vi "_Serial_Mark10-Control (Press Config).vi"(3 "FTS Operation state":T1="Start pressure control", 4 "Press Setting(lb)":dbl=10.0 min=0.0 max=160.0 step=0.01 format="%.2f", 5 "Serial Port":refnum<visa-resource-name>="COM5") -> (0 "Gauge Pressure(lb)":dbl min=0.0 max=160.0 step=0.01 format="%.2f", 1 "Communication is normal":bool=TRUE, 2 "Serial Port out":refnum<visa-resource-name>="COM5")   [LabVIEW 2015]
uses:
  Control-Operation State Mark10.ctl
panel:
  out "Number of fine tuning":u32
  in  "Speed-fine tuning(mm/min)":dbl=1.0
  in  "Speed-Low(mm/min)":dbl=4.0
  in  "Speed-Medium(mm/min)":dbl=60.0
  in  "Speed-High(mm/min)":dbl=250.0
  # "MARK10 Control of Press"
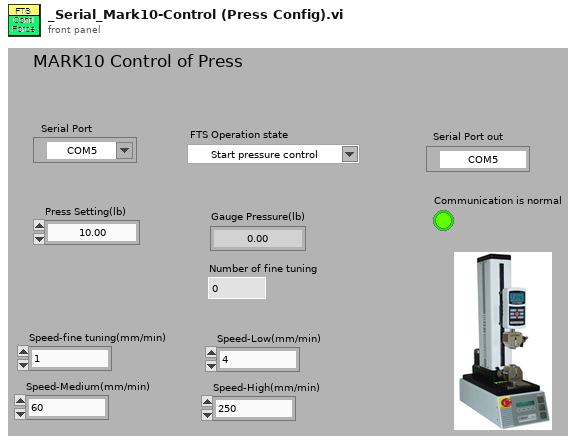
[diagram p1: front panel]
types:
  T1 = typedef "Control-Operation State Mark10.ctl" = string
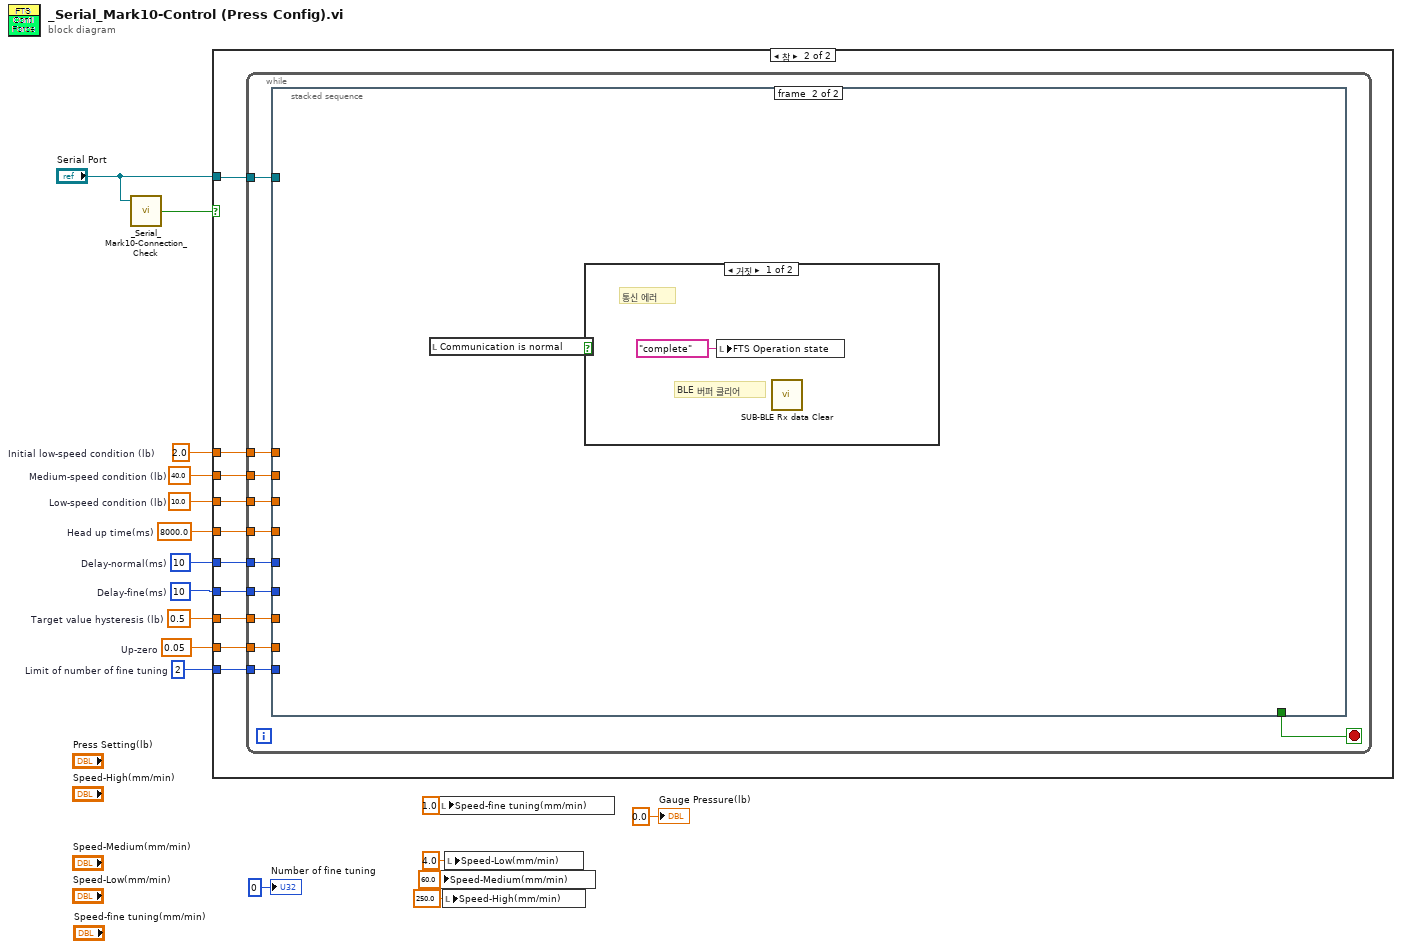
[diagram p0: block diagram]
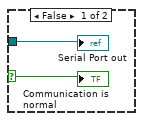
[diagram p2: hidden frame]
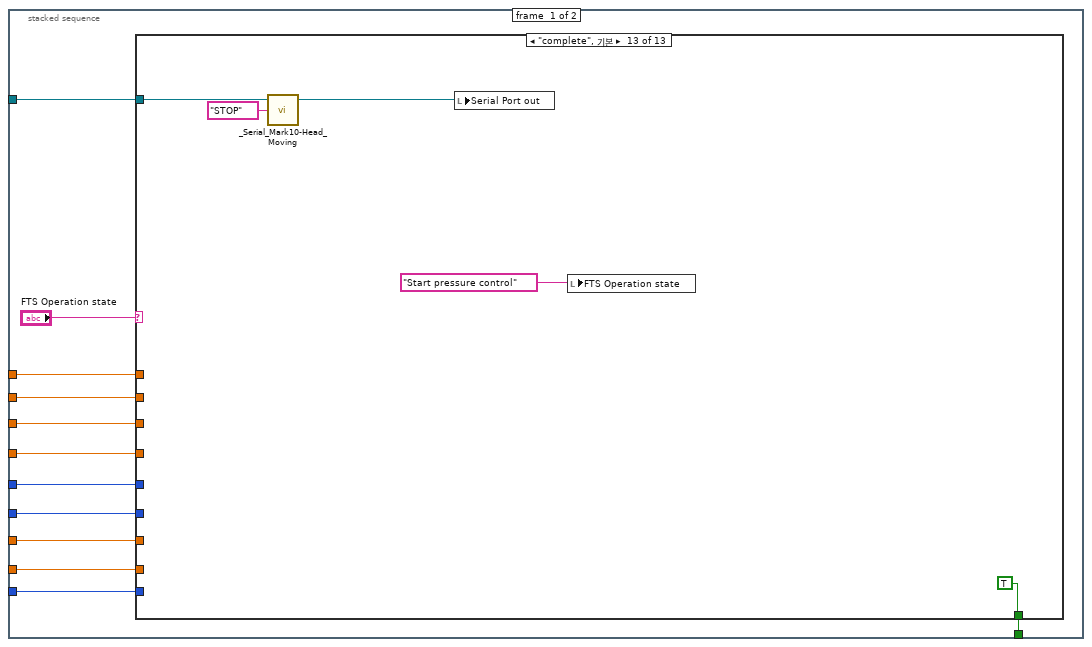
[diagram p3: hidden frame]
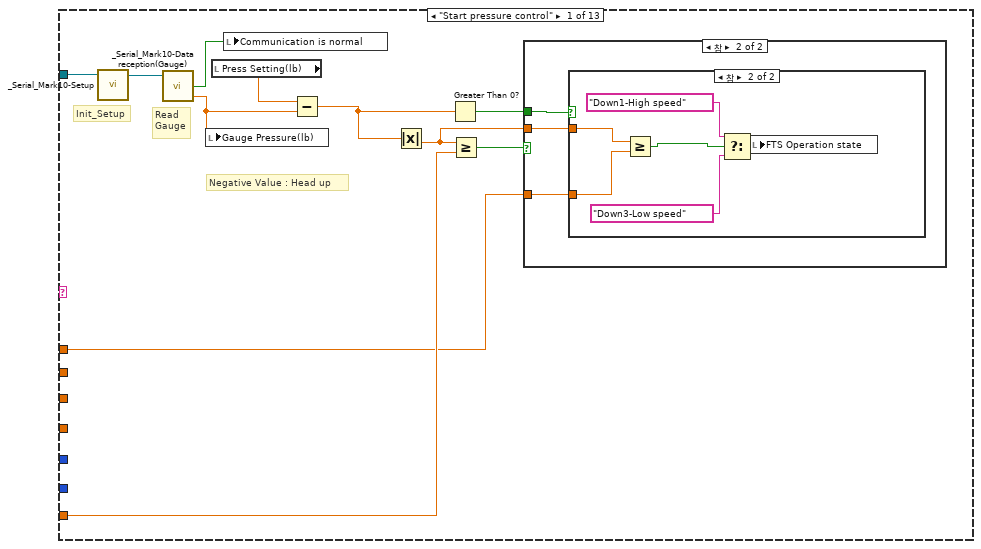
[diagram p4: hidden frame]
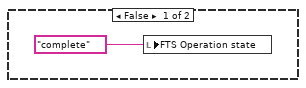
[diagram p5: hidden frame]
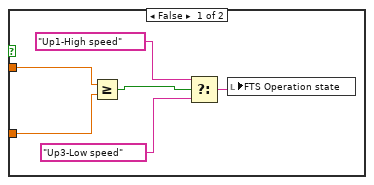
[diagram p6: hidden frame]
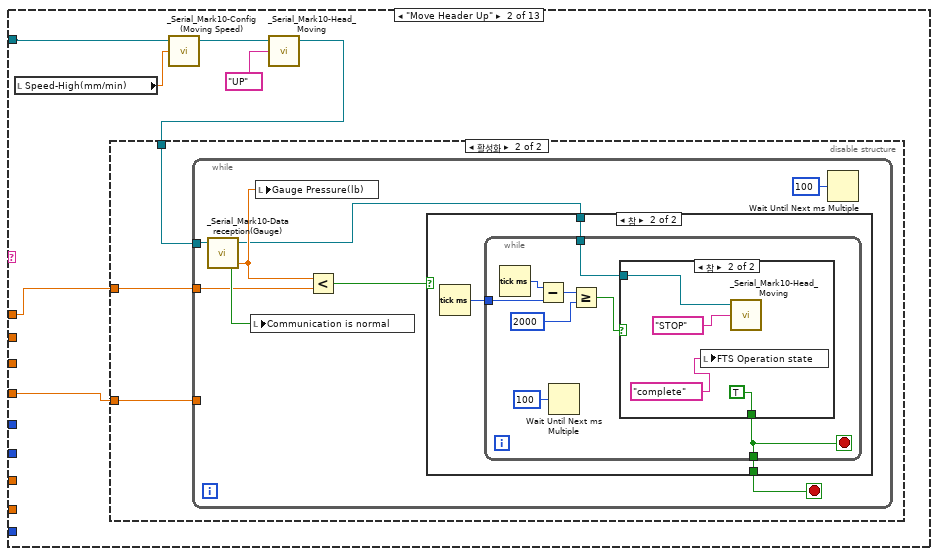
[diagram p7: hidden frame]
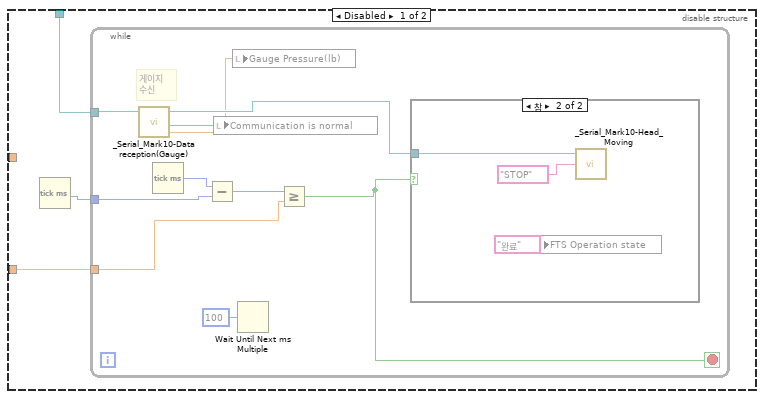
[diagram p8: hidden frame]
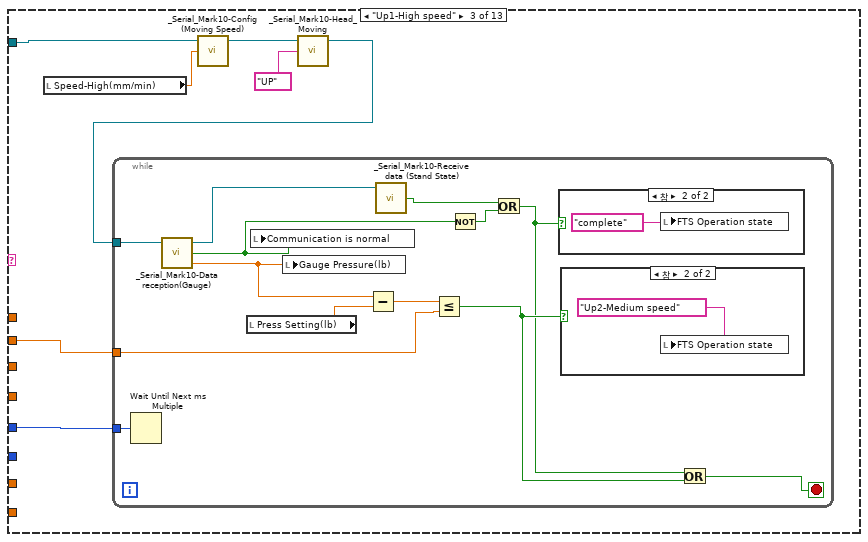
[diagram p12: hidden frame]
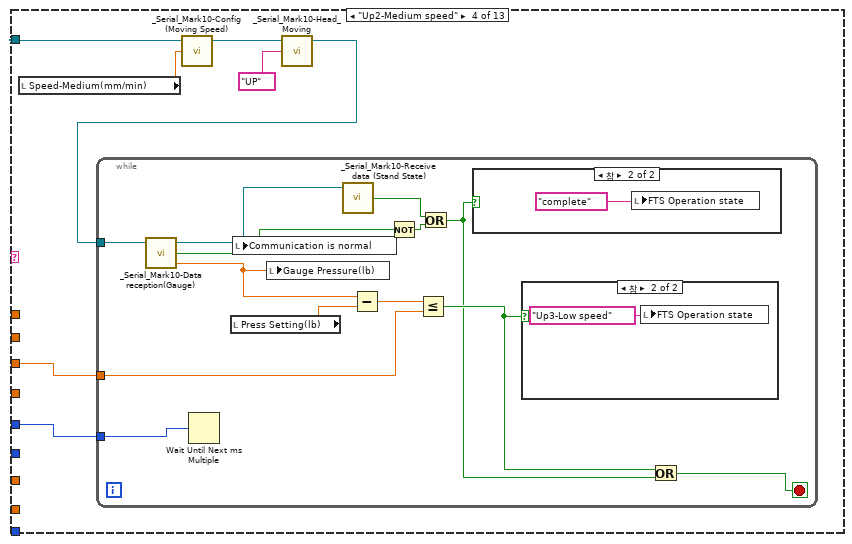
[diagram p15: hidden frame]
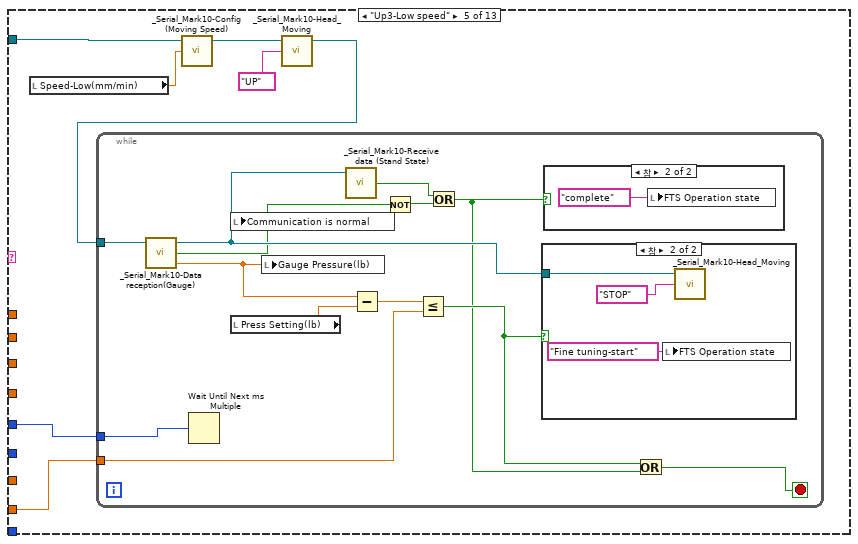
[diagram p18: hidden frame]
diagram:
  w1 = u32 2  # Limit of number of fine tuning
  w2 = 2.0  # Initial low-speed condition (lb)
  w3 = 0.05  # Up-zero
  w5 = 0.5  # Target value hysteresis (lb)
  w10 = u32 10  # Delay-fine(ms)
  w11 = u32 10  # Delay-normal(ms)
  w12 = 8000.0  # Head up time(ms)
  w13 = 10.0  # Low-speed condition (lb)
  w14 = 40.0  # Medium-speed condition (lb)
  n1 = call "_Serial_Mark10-Connection_Check.vi"("Serial Port"="Serial Port") -> ("Normal reception"=w15:bool)  [unwired: 3 in, 1 out]
  n2 = case shown="참" w15 {
    selector: w15 -> [w18 _]
    tunnel: "Serial Port" -> [w19 w29]
    tunnel: w14 -> [_ w28]
    tunnel: w13 -> [_ w27]
    tunnel: w12 -> [_ w26]
    tunnel: w11 -> [_ w25]
    tunnel: w10 -> [_ w24]
    tunnel: w5 -> [_ w23]
    tunnel: w3 -> [_ w22]
    tunnel: w2 -> [_ w21]
    tunnel: w1 -> [_ w20]
    frame False {
      "Communication is normal" <- w18
      "Serial Port out" <- w19
    }
    frame True {
      n3 = while {
        tunnel: w29 -> [w40]
        tunnel: w28 -> [w38]
        tunnel: w27 -> [w37]
        tunnel: w26 -> [w36]
        tunnel: w25 -> [w35]
        tunnel: w24 -> [w34]
        tunnel: w23 -> [w33]
        tunnel: w22 -> [w32]
        tunnel: w21 -> [w31]
        tunnel: w20 -> [w30]
        stop <- w39 stop-if-true
        n4 = stacked-sequence {
          tunnel: w40 -> [w52 _]
          tunnel: [w51 _] -> w39
          tunnel: w38 -> [w50 _]
          tunnel: w37 -> [w49 _]
          tunnel: w36 -> [w48 _]
          tunnel: w35 -> [w47 _]
          tunnel: w34 -> [w46 _]
          tunnel: w33 -> [w45 _]
          tunnel: w32 -> [w44 _]
          tunnel: w31 -> [w43 _]
          tunnel: w30 -> [w42 _]
          frame #0 {
            n5 = case shown="\"complete\", 기본" "FTS Operation state" {
              tunnel: w52 -> [w63 w82 w131 w153 w175 w202 w219 w240 w263 w291 w316 w342 w364]
              tunnel: [_ _ _ _ _ _ _ _ _ _ _ _ TRUE] -> w51
              tunnel: w50 -> [_ _ w130 _ _ w198 _ _ _ _ _ _ _]
              tunnel: w49 -> [_ _ _ w152 _ _ w218 _ _ _ _ _ _]
              tunnel: w48 -> [_ w81 _ _ _ _ _ _ _ _ _ _ _]
              tunnel: w47 -> [_ _ w129 w151 w174 w197 w217 w239 _ _ _ _ _]
              tunnel: w46 -> [_ _ _ _ _ _ _ _ _ w290 w315 _ _]
              tunnel: w45 -> [w54 _ _ _ _ _ _ _ w262 _ _ w341 _]
              tunnel: w44 -> [_ _ _ _ w173 _ _ _ _ _ w314 _ _]
              tunnel: w43 -> [w53 w80 _ _ _ _ _ _ _ _ _ _ _]
              tunnel: w42 -> [_ _ _ _ _ _ _ _ _ _ _ w340 _]
              frame "Start pressure control" {
                # "Negative Value : Head up"
                # "Read\nGauge"
                # "Init_Setup"
                n6 = call "_Serial_Mark10-Setup.vi"("Serial Port"=w63) -> ("VISA resource name out"=w62:refnum<visa-resource-name>)  [unwired: 4 in]
                n7 = call "_Serial_Mark10-Data reception(Gauge).vi"("Serial Port"=w62) -> ("data(lb)"=w60:dbl, "Normal reception"=w55:bool)  [unwired: 2 in, 1 out]
                n8 = local write "Gauge Pressure(lb)"(w60) -> ()
                n9 = local read "Press Setting(lb)"() -> (w61:dbl)
                n10 = local write "Communication is normal"(w55) -> ()
                n11 = Subtract(x=w61, y=w60) -> (x-y=w58:dbl)
                n12 = Absolute Value(x=w58) -> (abs(x)=w56:dbl)
                n13 = Greater Than 0?(x=w58) -> (x > 0?=w57:bool)
                n14 = Greater Or Equal?(x=w56, y=w54) -> (x >= y?=w59:bool)
                n15 = case shown="참" w59 {
                  tunnel: w57 -> [_ w67]
                  tunnel: w56 -> [_ w66]
                  tunnel: w53 -> [_ w65]
                  frame False {
                    n16 = local write "FTS Operation state"(T1 "complete" ("FTS 제어 상태")) -> ()
                  }
                  frame True {
                    n17 = case shown="참" w67 {
                      tunnel: w66 -> [w72 w79]
                      tunnel: w65 -> [w70 w76]
                      frame False {
                        n18 = Greater Or Equal?(x=w72, y=w70) -> (x >= y?=w73:bool)
                        n19 = Select(t=T1 "Up1-High speed" ("FTS 제어 상태"), s=w73, f=T1 "Up3-Low speed" ("FTS 제어 상태")) -> (s? t:f=w71:T1)
                        n20 = local write "FTS Operation state"(w71) -> ()
                      }
                      frame True {
                        n21 = Greater Or Equal?(x=w79, y=w76) -> (x >= y?=w78:bool)
                        n22 = Select(t=T1 "Down1-High speed" ("FTS 제어 상태"), s=w78, f=T1 "Down3-Low speed" ("FTS 제어 상태")) -> (s? t:f=w77:T1)
                        n23 = local write "FTS Operation state"(w77) -> ()
                      }
                    }
                  }
                }
              }
              frame "Move Header Up" {
                n24 = local read "Speed-High(mm/min)"() -> (w86:dbl)
                n25 = call "_Serial_Mark10-Config (Moving Speed).vi"("Speed(mm/min)"=w86, "Serial Port"=w82) -> ("VISA resource name out"=w84:refnum<visa-resource-name>)  [unwired: 3 in]
                n26 = call "_Serial_Mark10-Head_Moving.vi"("Operation Mode"="UP" ("동작 모드"), "Serial Port"=w84) -> ("VISA Resource name out"=w83:refnum<visa-resource-name>)  [unwired: 3 in]
                n27 = disable-structure shown="활성화" {
                  disable-tunnel: w83 -> [w89 w105]
                  disable-tunnel: w81 -> [w87 w104]
                  disable-tunnel: w80 -> [_ w103]
                  frame Disabled {
                    n28 = Tick Count (ms)() -> (millisecond timer value=w88:u32)
                    n29 = while {
                      tunnel: w89 -> [w99]
                      tunnel: w88 -> [w94]
                      tunnel: w87 -> [w92]
                      stop <- w91 stop-if-true
                      # "게이지\n수신"
                      n30 = call "_Serial_Mark10-Data reception(Gauge).vi"("Serial Port"=w99) -> ("data(lb)"=w96:dbl, "Normal reception"=w90:bool, "Serial Port out"=w98:refnum<visa-resource-name>)  [unwired: 2 in]
                      n31 = Tick Count (ms)() -> (millisecond timer value=w95:u32)
                      n32 = Subtract(x=w95, y=w94) -> (x-y=w93:u32)
                      n33 = local write "Communication is normal"(w90) -> ()
                      n34 = local write "Gauge Pressure(lb)"(w96) -> ()
                      n35 = Wait Until Next ms Multiple(millisecond multiple=u32 100 ("ms 배수")) -> ()  [unwired: 1 out]
                      n36 = Greater Or Equal?(x=w93, y=w92) -> (x >= y?=w91:bool)
                      n37 = case shown="참" w91 {
                        tunnel: w98 -> [_ w100]
                        frame False {
                        }
                        frame True {
                          n38 = local write "FTS Operation state"(T1 "완료" ("FTS 제어 상태")) -> ()
                          n39 = call "_Serial_Mark10-Head_Moving.vi"("Operation Mode"="STOP" ("동작 모드"), "Serial Port"=w100) -> ()  [unwired: 3 in, 1 out]
                        }
                      }
                    }
                  }
                  frame Enabled {
                    n40 = while {
                      tunnel: w105 -> [w113]
                      tunnel: w104 -> [_]
                      tunnel: w103 -> [w109]
                      stop <- w106 stop-if-true
                      n41 = call "_Serial_Mark10-Data reception(Gauge).vi"("Serial Port"=w113) -> ("data(lb)"=w110:dbl, "Normal reception"=w111:bool, "Serial Port out"=w107:refnum<visa-resource-name>)  [unwired: 2 in]
                      n42 = local write "Communication is normal"(w111) -> ()
                      n43 = local write "Gauge Pressure(lb)"(w110) -> ()
                      n44 = Less?(x=w110, y=w109) -> (x < y?=w108:bool)
                      n45 = case shown="참" w108 {
                        tunnel: w107 -> [_ w115]
                        tunnel: [_ w114] -> w106
                        frame False {
                        }
                        frame True {
                          n46 = Tick Count (ms)() -> (millisecond timer value=w116:u32)
                          n47 = while {
                            tunnel: w116 -> [w121]
                            tunnel: w115 -> [w118]
                            tunnel: [w117] -> w114
                            stop <- w117 stop-if-true
                            n48 = Tick Count (ms)() -> (millisecond timer value=w122:u32)
                            n49 = Subtract(x=w122, y=w121) -> (x-y=w123:u32)
                            n50 = Wait Until Next ms Multiple(millisecond multiple=u32 100 ("ms 배수")) -> ()  [unwired: 1 out]
                            n51 = Greater Or Equal?(x=w123, y=u32 2000) -> (x >= y?=w120:bool)
                            n52 = case shown="참" w120 {
                              tunnel: w118 -> [_ w127]
                              tunnel: [_ TRUE] -> w117
                              frame False {
                              }
                              frame True {
                                n53 = local write "FTS Operation state"(T1 "complete" ("FTS 제어 상태")) -> ()
                                n54 = call "_Serial_Mark10-Head_Moving.vi"("Operation Mode"="STOP" ("동작 모드"), "Serial Port"=w127) -> ()  [unwired: 3 in, 1 out]
                              }
                            }
                          }
                        }
                      }
                      n55 = Wait Until Next ms Multiple(millisecond multiple=u32 100 ("ms 배수")) -> ()  [unwired: 1 out]
                    }
                  }
                }
              }
              frame "Up1-High speed" {
                n56 = local read "Speed-High(mm/min)"() -> (w135:dbl)
                n57 = call "_Serial_Mark10-Config (Moving Speed).vi"("Speed(mm/min)"=w135, "Serial Port"=w131) -> ("VISA resource name out"=w133:refnum<visa-resource-name>)  [unwired: 3 in]
                n58 = call "_Serial_Mark10-Head_Moving.vi"("Operation Mode"="UP" ("동작 모드"), "Serial Port"=w133) -> ("VISA Resource name out"=w132:refnum<visa-resource-name>)  [unwired: 3 in]
                n59 = while {
                  tunnel: w132 -> [w148]
                  tunnel: w130 -> [w144]
                  tunnel: w129 -> [w143]
                  stop <- w140 stop-if-true
                  n60 = Wait Until Next ms Multiple(millisecond multiple=w143) -> ()  [unwired: 1 out]
                  n61 = call "_Serial_Mark10-Data reception(Gauge).vi"("Serial Port"=w148) -> ("data(lb)"=w145:dbl, "Normal reception"=w136:bool, "Serial Port out"=w142:refnum<visa-resource-name>)  [unwired: 2 in]
                  n62 = local read "Press Setting(lb)"() -> (w147:dbl)
                  n63 = local write "Communication is normal"(w136) -> ()
                  n64 = local write "Gauge Pressure(lb)"(w145) -> ()
                  n65 = Subtract(x=w145, y=w147) -> (x-y=w146:dbl)
                  n66 = call "_Serial_Mark10-Receive data (Stand State).vi"("Serial Port"=w142) -> ("Motor Stop State"=w138:bool)  [unwired: 3 in, 1 out]
                  n67 = Less Or Equal?(x=w146, y=w144) -> (x <= y?=w141:bool)
                  n68 = Not(x=w136) -> (.not. x?=w137:bool)
                  n69 = Or(x=w138, y=w137) -> (x .or. y?=w139:bool)
                  n70 = case shown="참" w139 {
                    frame False {
                    }
                    frame True {
                      n71 = local write "FTS Operation state"(T1 "complete" ("FTS 제어 상태")) -> ()
                    }
                  }
                  n72 = case shown="참" w141 {
                    frame False {
                    }
                    frame True {
                      n73 = local write "FTS Operation state"(T1 "Up2-Medium speed" ("FTS 제어 상태")) -> ()
                    }
                  }
                  n74 = Or(x=w139, y=w141) -> (x .or. y?=w140:bool)
                }
              }
              frame "Up2-Medium speed" {
                n75 = local read "Speed-Medium(mm/min)"() -> (w157:dbl)
                n76 = call "_Serial_Mark10-Config (Moving Speed).vi"("Speed(mm/min)"=w157, "Serial Port"=w153) -> ("VISA resource name out"=w155:refnum<visa-resource-name>)  [unwired: 3 in]
                n77 = call "_Serial_Mark10-Head_Moving.vi"("Operation Mode"="UP" ("동작 모드"), "Serial Port"=w155) -> ("VISA Resource name out"=w154:refnum<visa-resource-name>)  [unwired: 3 in]
                n78 = while {
                  tunnel: w154 -> [w170]
                  tunnel: w152 -> [w166]
                  tunnel: w151 -> [w165]
                  stop <- w162 stop-if-true
                  n79 = call "_Serial_Mark10-Data reception(Gauge).vi"("Serial Port"=w170) -> ("data(lb)"=w167:dbl, "Normal reception"=w158:bool, "Serial Port out"=w164:refnum<visa-resource-name>)  [unwired: 2 in]
                  n80 = Wait Until Next ms Multiple(millisecond multiple=w165) -> ()  [unwired: 1 out]
                  n81 = local read "Press Setting(lb)"() -> (w169:dbl)
                  n82 = local write "Communication is normal"(w158) -> ()
                  n83 = local write "Gauge Pressure(lb)"(w167) -> ()
                  n84 = call "_Serial_Mark10-Receive data (Stand State).vi"("Serial Port"=w164) -> ("Motor Stop State"=w160:bool)  [unwired: 3 in, 1 out]
                  n85 = Subtract(x=w167, y=w169) -> (x-y=w168:dbl)
                  n86 = Not(x=w158) -> (.not. x?=w161:bool)
                  n87 = Less Or Equal?(x=w168, y=w166) -> (x <= y?=w163:bool)
                  n88 = Or(x=w160, y=w161) -> (x .or. y?=w159:bool)
                  n89 = case shown="참" w159 {
                    frame False {
                    }
                    frame True {
                      n90 = local write "FTS Operation state"(T1 "complete" ("FTS 제어 상태")) -> ()
                    }
                  }
                  n91 = case shown="참" w163 {
                    frame False {
                    }
                    frame True {
                      n92 = local write "FTS Operation state"(T1 "Up3-Low speed" ("FTS 제어 상태")) -> ()
                    }
                  }
                  n93 = Or(x=w163, y=w159) -> (x .or. y?=w162:bool)
                }
              }
              frame "Up3-Low speed" {
                n94 = local read "Speed-Low(mm/min)"() -> (w179:dbl)
                n95 = call "_Serial_Mark10-Config (Moving Speed).vi"("Speed(mm/min)"=w179, "Serial Port"=w175) -> ("VISA resource name out"=w177:refnum<visa-resource-name>)  [unwired: 3 in]
                n96 = call "_Serial_Mark10-Head_Moving.vi"("Operation Mode"="UP" ("동작 모드"), "Serial Port"=w177) -> ("VISA Resource name out"=w176:refnum<visa-resource-name>)  [unwired: 3 in]
                n97 = while {
                  tunnel: w176 -> [w192]
                  tunnel: w174 -> [w188]
                  tunnel: w173 -> [w180]
                  stop <- w185 stop-if-true
                  n98 = call "_Serial_Mark10-Data reception(Gauge).vi"("Serial Port"=w192) -> ("data(lb)"=w189:dbl, "Normal reception"=w184:bool, "Serial Port out"=w187:refnum<visa-resource-name>)  [unwired: 2 in]
                  n99 = Wait Until Next ms Multiple(millisecond multiple=w188) -> ()  [unwired: 1 out]
                  n100 = local write "Communication is normal"(w184) -> ()
                  n101 = local read "Press Setting(lb)"() -> (w191:dbl)
                  n102 = local write "Gauge Pressure(lb)"(w189) -> ()
                  n103 = call "_Serial_Mark10-Receive data (Stand State).vi"("Serial Port"=w187) -> ("Motor Stop State"=w182:bool)  [unwired: 3 in, 1 out]
                  n104 = Subtract(x=w189, y=w191) -> (x-y=w190:dbl)
                  n105 = Not(x=w184) -> (.not. x?=w183:bool)
                  n106 = Less Or Equal?(x=w190, y=w180) -> (x <= y?=w186:bool)
                  n107 = Or(x=w182, y=w183) -> (x .or. y?=w181:bool)
                  n108 = case shown="참" w186 {
                    tunnel: w187 -> [_ w195]
                    frame False {
                    }
                    frame True {
                      n109 = local write "FTS Operation state"(T1 "Fine tuning-start" ("FTS Operation state")) -> ()
                      n110 = call "_Serial_Mark10-Head_Moving.vi"("Operation Mode"="STOP" ("동작 모드"), "Serial Port"=w195) -> ()  [unwired: 3 in, 1 out]
                    }
                  }
                  n111 = case shown="참" w181 {
                    frame False {
                    }
                    frame True {
                      n112 = local write "FTS Operation state"(T1 "complete" ("FTS Operation state")) -> ()
                    }
                  }
                  n113 = Or(x=w186, y=w181) -> (x .or. y?=w185:bool)
                }
              }
              frame "Down1-High speed" {
                n114 = local read "Speed-High(mm/min)"() -> (w203:dbl)
                n115 = call "_Serial_Mark10-Config (Moving Speed).vi"("Speed(mm/min)"=w203, "Serial Port"=w202) -> ("VISA resource name out"=w200:refnum<visa-resource-name>)  [unwired: 3 in]
                n116 = call "_Serial_Mark10-Head_Moving.vi"("Operation Mode"="DOWN" ("동작 모드"), "Serial Port"=w200) -> ("VISA Resource name out"=w199:refnum<visa-resource-name>)  [unwired: 3 in]
                n117 = while {
                  tunnel: w199 -> [w214]
                  tunnel: w198 -> [_]
                  tunnel: w197 -> [w211]
                  stop <- w208 stop-if-true
                  n118 = call "_Serial_Mark10-Data reception(Gauge).vi"("Serial Port"=w214) -> ("data(lb)"=w213:dbl, "Normal reception"=w207:bool, "Serial Port out"=w210:refnum<visa-resource-name>)  [unwired: 2 in]
                  n119 = Wait Until Next ms Multiple(millisecond multiple=w211) -> ()  [unwired: 1 out]
                  n120 = local write "Communication is normal"(w207) -> ()
                  n121 = local write "Gauge Pressure(lb)"(w213) -> ()
                  n122 = Greater Or Equal?(x=w213, y=1.0) -> (x >= y?=w209:bool)
                  n123 = call "_Serial_Mark10-Receive data (Stand State).vi"("Serial Port"=w210) -> ("Motor Stop State"=w205:bool)  [unwired: 3 in, 1 out]
                  n124 = Not(x=w207) -> (.not. x?=w206:bool)
                  n125 = Or(x=w205, y=w206) -> (x .or. y?=w204:bool)
                  n126 = case shown="참" w209 {
                    frame False {
                    }
                    frame True {
                      n127 = local write "FTS Operation state"(T1 "Down2-Medium speed" ("FTS Operation state")) -> ()
                    }
                  }
                  n128 = case shown="참" w204 {
                    frame False {
                    }
                    frame True {
                      n129 = local write "FTS Operation state"(T1 "complete" ("FTS Operation state")) -> ()
                    }
                  }
                  n130 = Or(x=w204, y=w209) -> (x .or. y?=w208:bool)
                }
              }
              frame "Down2-Medium speed" {
                n131 = local read "Speed-Medium(mm/min)"() -> (w223:dbl)
                n132 = call "_Serial_Mark10-Config (Moving Speed).vi"("Speed(mm/min)"=w223, "Serial Port"=w219) -> ("VISA resource name out"=w221:refnum<visa-resource-name>)  [unwired: 3 in]
                n133 = call "_Serial_Mark10-Head_Moving.vi"("Operation Mode"="DOWN" ("동작 모드"), "Serial Port"=w221) -> ("VISA Resource name out"=w220:refnum<visa-resource-name>)  [unwired: 3 in]
                n134 = while {
                  tunnel: w220 -> [w236]
                  tunnel: w218 -> [w232]
                  tunnel: w217 -> [w231]
                  stop <- w228 stop-if-true
                  n135 = call "_Serial_Mark10-Data reception(Gauge).vi"("Serial Port"=w236) -> ("data(lb)"=w233:dbl, "Normal reception"=w227:bool, "Serial Port out"=w230:refnum<visa-resource-name>)  [unwired: 2 in]
                  n136 = Wait Until Next ms Multiple(millisecond multiple=w231) -> ()  [unwired: 1 out]
                  n137 = local write "Communication is normal"(w227) -> ()
                  n138 = local read "Press Setting(lb)"() -> (w235:dbl)
                  n139 = local write "Gauge Pressure(lb)"(w233) -> ()
                  n140 = call "_Serial_Mark10-Receive data (Stand State).vi"("Serial Port"=w230) -> ("Motor Stop State"=w225:bool)  [unwired: 3 in, 1 out]
                  n141 = Subtract(x=w235, y=w233) -> (x-y=w234:dbl)
                  n142 = Not(x=w227) -> (.not. x?=w226:bool)
                  n143 = Less Or Equal?(x=w234, y=w232) -> (x <= y?=w229:bool)
                  n144 = Or(x=w225, y=w226) -> (x .or. y?=w224:bool)
                  n145 = case shown="참" w229 {
                    frame False {
                    }
                    frame True {
                      n146 = local write "FTS Operation state"(T1 "Down3-Low speed" ("FTS Operation state")) -> ()
                    }
                  }
                  n147 = case shown="참" w224 {
                    frame False {
                    }
                    frame True {
                      n148 = local write "FTS Operation state"(T1 "complete" ("FTS Operation state")) -> ()
                    }
                  }
                  n149 = Or(x=w229, y=w224) -> (x .or. y?=w228:bool)
                }
              }
              frame "Down3-Low speed" {
                n150 = local read "Speed-Low(mm/min)"() -> (w244:dbl)
                n151 = call "_Serial_Mark10-Config (Moving Speed).vi"("Speed(mm/min)"=w244, "Serial Port"=w240) -> ("VISA resource name out"=w242:refnum<visa-resource-name>)  [unwired: 3 in]
                n152 = call "_Serial_Mark10-Head_Moving.vi"("Operation Mode"="DOWN" ("동작 모드"), "Serial Port"=w242) -> ("VISA Resource name out"=w241:refnum<visa-resource-name>)  [unwired: 3 in]
                n153 = while {
                  tunnel: w241 -> [w257]
                  tunnel: w239 -> [w253]
                  stop <- w251 stop-if-true
                  n154 = call "_Serial_Mark10-Data reception(Gauge).vi"("Serial Port"=w257) -> ("data(lb)"=w254:dbl, "Normal reception"=w245:bool, "Serial Port out"=w250:refnum<visa-resource-name>)  [unwired: 2 in]
                  n155 = Wait Until Next ms Multiple(millisecond multiple=w253) -> ()  [unwired: 1 out]
                  n156 = local write "Communication is normal"(w245) -> ()
                  n157 = local read "Press Setting(lb)"() -> (w256:dbl)
                  n158 = local write "Gauge Pressure(lb)"(w254) -> ()
                  n159 = Subtract(x=w256, y=w254) -> (x-y=w255:dbl)
                  n160 = call "_Serial_Mark10-Receive data (Stand State).vi"("Serial Port"=w250) -> ("Motor Stop State"=w248:bool, "Serial Port out"=w249:refnum<visa-resource-name>)  [unwired: 3 in]
                  n161 = Less Or Equal To 0?(x=w255) -> (x <= 0?=w252:bool)
                  n162 = Not(x=w245) -> (.not. x?=w247:bool)
                  n163 = Or(x=w248, y=w247) -> (x .or. y?=w246:bool)
                  n164 = case shown="참" w252 {
                    tunnel: w249 -> [_ w260]
                    frame False {
                    }
                    frame True {
                      n165 = local write "FTS Operation state"(T1 "Fine tuning-start" ("FTS Operation state")) -> ()
                      n166 = call "_Serial_Mark10-Head_Moving.vi"("Operation Mode"="STOP" ("동작 모드"), "Serial Port"=w260) -> ()  [unwired: 3 in, 1 out]
                    }
                  }
                  n167 = case shown="참" w246 {
                    frame False {
                    }
                    frame True {
                      n168 = local write "FTS Operation state"(T1 "complete" ("FTS Operation state")) -> ()
                    }
                  }
                  n169 = Or(x=w252, y=w246) -> (x .or. y?=w251:bool)
                }
              }
              frame "Fine tuning-start" {
                n170 = stacked-sequence {
                  tunnel: w263 -> [w266 w284]
                  tunnel: w262 -> [_ w281]
                  frame #0 {
                    w264 = u32 500  # Timeout(ms)
                    # "Wait for the pressure to stabilize."
                    n171 = Tick Count (ms)() -> (millisecond timer value=w265:u32)
                    n172 = while {
                      tunnel: w266 -> [w275]
                      tunnel: w265 -> [w271]
                      tunnel: w264 -> [w269]
                      stop <- w268 stop-if-true
                      n173 = call "_Serial_Mark10-Data reception(Gauge).vi"("Serial Port"=w275) -> ("data(lb)"=w273:dbl, "Normal reception"=w267:bool)  [unwired: 2 in, 1 out]
                      n174 = Tick Count (ms)() -> (millisecond timer value=w272:u32)
                      n175 = local write "Communication is normal"(w267) -> ()
                      n176 = Subtract(x=w272, y=w271) -> (x-y=w270:u32)
                      n177 = local write "Gauge Pressure(lb)"(w273) -> ()
                      n178 = Wait Until Next ms Multiple(millisecond multiple=u32 50 ("ms 배수")) -> ()  [unwired: 1 out]
                      n179 = Greater Or Equal?(x=w270, y=w269) -> (x >= y?=w268:bool)
                    }
                  }
                  frame #1 {
                    n180 = call "_Serial_Mark10-Data reception(Gauge).vi"("Serial Port"=w284) -> ("data(lb)"=w285:dbl, "Normal reception"=w283:bool)  [unwired: 2 in, 1 out]
                    n181 = local write "Communication is normal"(w283) -> ()
                    n182 = local write "Gauge Pressure(lb)"(w285) -> ()
                    n183 = local read "Press Setting(lb)"() -> (w286:dbl)
                    n184 = Subtract(x=w286, y=w285) -> (x-y=w282:dbl)
                    n185 = Multiply(x=w281, y=-1.0) -> (x*y=w280:dbl)
                    n186 = Greater Or Equal?(x=w282, y=w281) -> (x >= y?=w277:bool)
                    n187 = Less Or Equal?(x=w282, y=w280) -> (x <= y?=w278:bool)
                    n188 = Or(x=w278, y=w277) -> (x .or. y?=w276:bool)
                    n189 = case shown="참" w277 {
                      frame False {
                      }
                      frame True {
                        n190 = local write "FTS Operation state"(T1 "Fine tuning-down" ("FTS Operation state")) -> ()
                      }
                    }
                    n191 = case shown="참" w278 {
                      frame False {
                      }
                      frame True {
                        n192 = local write "FTS Operation state"(T1 "Fine tuning-up" ("FTS Operation state")) -> ()
                      }
                    }
                    n193 = case shown="거짓" w276 {
                      frame False {
                        n194 = local write "FTS Operation state"(T1 "Fine tuning-end" ("FTS Operation state")) -> ()
                      }
                      frame True {
                      }
                    }
                  }
                }
              }
              frame "Fine tuning-down" {
                n195 = local read "Speed-fine tuning(mm/min)"() -> (w295:dbl)
                n196 = call "_Serial_Mark10-Config (Moving Speed).vi"("Speed(mm/min)"=w295, "Serial Port"=w291) -> ("VISA resource name out"=w293:refnum<visa-resource-name>)  [unwired: 3 in]
                n197 = call "_Serial_Mark10-Head_Moving.vi"("Operation Mode"="DOWN" ("동작 모드"), "Serial Port"=w293) -> ("VISA Resource name out"=w292:refnum<visa-resource-name>)  [unwired: 3 in]
                n198 = while {
                  tunnel: w292 -> [w308]
                  tunnel: w290 -> [w302]
                  stop <- w303 stop-if-true
                  n199 = call "_Serial_Mark10-Data reception(Gauge).vi"("Serial Port"=w308) -> ("data(lb)"=w305:dbl, "Normal reception"=w296:bool, "Serial Port out"=w301:refnum<visa-resource-name>)  [unwired: 2 in]
                  n200 = local write "Communication is normal"(w296) -> ()
                  n201 = local read "Press Setting(lb)"() -> (w307:dbl)
                  n202 = local write "Gauge Pressure(lb)"(w305) -> ()
                  n203 = call "_Serial_Mark10-Receive data (Stand State).vi"("Serial Port"=w301) -> ("Motor Stop State"=w298:bool, "Serial Port out"=w300:refnum<visa-resource-name>)  [unwired: 3 in]
                  n204 = Subtract(x=w307, y=w305) -> (x-y=w306:dbl)
                  n205 = Not(x=w296) -> (.not. x?=w299:bool)
                  n206 = Less Or Equal To 0?(x=w306) -> (x <= 0?=w304:bool)
                  n207 = Or(x=w298, y=w299) -> (x .or. y?=w297:bool)
                  n208 = case shown="참" w304 {
                    tunnel: w300 -> [_ w312]
                    tunnel: w302 -> [w310 _]
                    frame False {
                      n209 = Wait Until Next ms Multiple(millisecond multiple=w310) -> ()  [unwired: 1 out]
                    }
                    frame True {
                      n210 = local write "FTS Operation state"(T1 "Fine tuning-end" ("FTS Operation state")) -> ()
                      n211 = call "_Serial_Mark10-Head_Moving.vi"("Operation Mode"="STOP" ("동작 모드"), "Serial Port"=w312) -> ()  [unwired: 3 in, 1 out]
                    }
                  }
                  n212 = case shown="참" w297 {
                    frame False {
                    }
                    frame True {
                      n213 = local write "FTS Operation state"(T1 "complete" ("FTS Operation state")) -> ()
                    }
                  }
                  n214 = Or(x=w304, y=w297) -> (x .or. y?=w303:bool)
                }
              }
              frame "Fine tuning-up" {
                n215 = local read "Speed-Low(mm/min)"() -> (w320:dbl)
                n216 = call "_Serial_Mark10-Config (Moving Speed).vi"("Speed(mm/min)"=w320, "Serial Port"=w316) -> ("VISA resource name out"=w318:refnum<visa-resource-name>)  [unwired: 3 in]
                n217 = call "_Serial_Mark10-Head_Moving.vi"("Operation Mode"="UP" ("동작 모드"), "Serial Port"=w318) -> ("VISA Resource name out"=w317:refnum<visa-resource-name>)  [unwired: 3 in]
                n218 = while {
                  tunnel: w317 -> [w334]
                  tunnel: w315 -> [w328]
                  tunnel: w314 -> [w321]
                  stop <- w329 stop-if-true
                  n219 = call "_Serial_Mark10-Data reception(Gauge).vi"("Serial Port"=w334) -> ("data(lb)"=w331:dbl, "Normal reception"=w323:bool, "Serial Port out"=w327:refnum<visa-resource-name>)  [unwired: 2 in]
                  n220 = local write "Communication is normal"(w323) -> ()
                  n221 = local read "Press Setting(lb)"() -> (w333:dbl)
                  n222 = local write "Gauge Pressure(lb)"(w331) -> ()
                  n223 = call "_Serial_Mark10-Receive data (Stand State).vi"("Serial Port"=w327) -> ("Motor Stop State"=w325:bool, "Serial Port out"=w326:refnum<visa-resource-name>)  [unwired: 3 in]
                  n224 = Subtract(x=w331, y=w333) -> (x-y=w332:dbl)
                  n225 = Not(x=w323) -> (.not. x?=w324:bool)
                  n226 = Less Or Equal?(x=w332, y=w321) -> (x <= y?=w330:bool)
                  n227 = Or(x=w325, y=w324) -> (x .or. y?=w322:bool)
                  n228 = case shown="참" w322 {
                    frame False {
                    }
                    frame True {
                      n229 = local write "FTS Operation state"(T1 "complete" ("FTS Operation state")) -> ()
                    }
                  }
                  n230 = case shown="참" w330 {
                    tunnel: w326 -> [_ w338]
                    tunnel: w328 -> [w336 _]
                    frame False {
                      n231 = Wait Until Next ms Multiple(millisecond multiple=w336) -> ()  [unwired: 1 out]
                    }
                    frame True {
                      n232 = local write "FTS Operation state"(T1 "Fine tuning-end" ("FTS Operation state")) -> ()
                      n233 = call "_Serial_Mark10-Head_Moving.vi"("Operation Mode"="STOP" ("동작 모드"), "Serial Port"=w338) -> ()  [unwired: 3 in, 1 out]
                    }
                  }
                  n234 = Or(x=w330, y=w322) -> (x .or. y?=w329:bool)
                }
              }
              frame "Fine tuning-end" {
                n235 = stacked-sequence {
                  tunnel: w342 -> [_ w347]
                  tunnel: w341 -> [_ w345]
                  tunnel: w340 -> [_ w344]
                  frame #0 {
                    n236 = Wait Until Next ms Multiple(millisecond multiple=u32 1000 ("ms 배수")) -> ()  [unwired: 1 out]
                  }
                  frame #1 {
                    n237 = call "_Serial_Mark10-Data reception(Gauge).vi"("Serial Port"=w347) -> ("data(lb)"=w351:dbl, "Normal reception"=w346:bool)  [unwired: 2 in, 1 out]
                    n238 = local write "Communication is normal"(w346) -> ()
                    n239 = local write "Gauge Pressure(lb)"(w351) -> ()
                    n240 = local read "Press Setting(lb)"() -> (w352:dbl)
                    n241 = Subtract(x=w352, y=w351) -> (x-y=w349:dbl)
                    n242 = Absolute Value(x=w349) -> (abs(x)=w348:dbl)
                    n243 = Greater Or Equal?(x=w348, y=w345) -> (x >= y?=w350:bool)
                    n244 = case shown="참" w350 {
                      tunnel: w344 -> [w353 _]
                      frame False {
                        # "Reaching the target"
                        n245 = local read "Number of fine tuning"() -> (w356:u32)
                        n246 = Increment(x=w356) -> (x+1=w355:u32)
                        n247 = Greater Or Equal?(x=w355, y=w353) -> (x >= y?=w354:bool)
                        n248 = case shown="참" w354 {
                          frame False {
                            n249 = local write "FTS Operation state"(T1 "Fine tuning-start" ("FTS Operation state")) -> ()
                          }
                          frame True {
                            n250 = local write "FTS Operation state"(T1 "complete" ("FTS Operation state")) -> ()
                          }
                        }
                        n251 = local write "Number of fine tuning"(w355) -> ()
                      }
                      frame True {
                        n252 = local write "Number of fine tuning"(u32 0 ("미세조정 횟수")) -> ()
                        n253 = local write "FTS Operation state"(T1 "Fine tuning-start" ("FTS Operation state")) -> ()
                      }
                    }
                  }
                }
              }
              frame "complete", Default {
                n254 = call "_Serial_Mark10-Head_Moving.vi"("Operation Mode"="STOP" ("동작 모드"), "Serial Port"=w364) -> ("VISA Resource name out"=w362:refnum<visa-resource-name>)  [unwired: 3 in]
                n255 = local write "Serial Port out"(w362) -> ()
                n256 = local write "FTS Operation state"(T1 "Start pressure control" ("FTS 제어 상태")) -> ()
              }
            }
          }
          frame #1 {
            n257 = local read "Communication is normal"() -> (w366:bool)
            n258 = case shown="거짓" w366 {
              frame False {
                # "BLE 버퍼 클리어"
                # "통신 에러"
                n259 = local write "FTS Operation state"(T1 "complete" ("FTS Operation state")) -> ()
                n260 = call "SUB-BLE Rx data Clear.vi"() -> ()  [unwired: 6 in]
              }
              frame True {
              }
            }
          }
        }
      }
    }
  }
  n261 = local write "Speed-Medium(mm/min)"(60.0 ("속도-중속(mm/min)")) -> ()
  n262 = local write "Speed-fine tuning(mm/min)"(1.0 ("속도-미세조정(mm/min)")) -> ()
  n263 = local write "Speed-High(mm/min)"(250.0 ("속도-고속(mm/min)")) -> ()
  n264 = local write "Speed-Low(mm/min)"(4.0 ("속도-저속(mm/min)")) -> ()
  "Gauge Pressure(lb)" <- 0.0 ("게이지 압력(lb)")
  "Number of fine tuning" <- u32 0 ("지연시간-미세(ms)")
